vi "Cov_Temp.vi"(11 "Input x":dbl) -> (3 "Temperature":dbl)   [LabVIEW 2011]
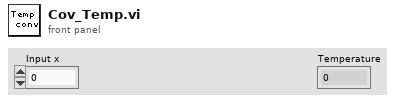
[diagram p1: front panel]
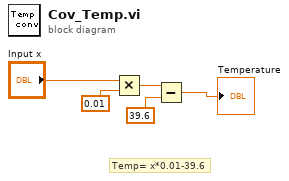
[diagram p0: block diagram]
diagram:
  # "Temp= x*0.01-39.6"
  n1 = Multiply(x="Input x", y=0.01) -> (x*y=w5:dbl)
  n2 = Subtract(x=w5, y=39.6) -> (x-y=→"Temperature":dbl)
